vi "2 - Real API list + loop.vi"() -> ()   [LabVIEW 2020]
uses:
  client/client.lvlib
panel:
  out "Array":string[](array[string])
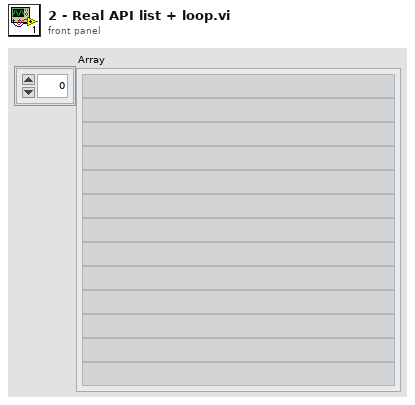
[diagram p1: front panel]
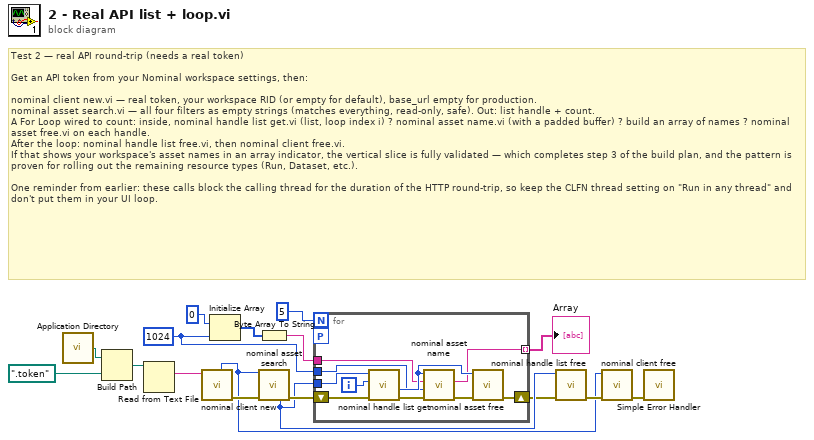
[diagram p0: block diagram]
diagram:
  w7 = 1024
  # "Test 2 — real API round-trip (needs a real token)\n\nGet an API token from your Nominal workspace settings, then:\n\nnominal client new.vi — real token, your workspace RID (or empty for default), base_url empty for production.\nnominal asset search.vi — all four filters as empty strings (matches everything, read-only, safe). Out: list handle + count.\nA For Loop wired to count: inside, nominal handle list get.vi (list, loop index i) ? nominal asset name.vi (with a padded buffer) ? build an array of names ? nominal asset free.vi on each handle.\nAfter the loop: nominal handle list free.vi, then nominal client free.vi.\nIf that shows your workspace's asset names in an array indicator, the vertical slice is fully validated — which completes step 3 of the build plan, and the pattern is proven for rolling out the remaining resource types (Run, Dataset, etc.).\n\nOne reminder from earlier: these calls block the calling thread for the duration of the HTTP round-trip, so keep the CLFN thread setting on \"Run in any thread\" and don't put them in your UI loop."
  n1 = call <vilib>:"Application Directory.vi"() -> ("Application Directory"=w5:path)
  n2 = Build Path(base path=w5, name or relative path=path ".token") -> (appended path=w3:path)
  n3 = Read from Text File(file (use dialog)=w3) -> (text=w2:string)  [unwired: 3 in, 3 out]
  n4 = call "nominal client new.vi"("token"=w2) -> ("error out"=w16:errorcluster, "out_client out"=w12:i32)  [unwired: 8 in, 1 out]
  n5 = Initialize Array(u8 0, w7) -> (w9:u8[])
  n6 = Byte Array To String(unsigned byte array=w9) -> (string=w8:string)
  n7 = call "nominal asset search.vi"("client"=w12, "error in (no error)"=w16) -> ("out_list out"=w15:i32, "error out"=w17:errorcluster)  [unwired: 10 in, 2 out]
  n8 = for {
    N: 5 -> [_]
    tunnel: w15 -> [w27]
    shift-right: [w21] -> w14
    shift-left: w17 -> [w22]
    tunnel: w8 -> [w20]
    tunnel: w7 -> [w19]
    tunnel: [w18] -> w6 mode=indexing
    workers-P: _ -> [_]
    i -> [w25]
    n9 = call "nominal handle list get.vi"("error in (no error)"=w22, "index"=w25, "list"=w27) -> ("error out"=w23:errorcluster, "out_handle out"=w26:i32)  [unwired: 6 in, 1 out]
    n10 = call "nominal asset name.vi"("error in (no error)"=w23, "cap"=w19, "buf"=w20, "asset"=w26) -> ("error out"=w24:errorcluster, "buf out"=w18:string)  [unwired: 4 in, 2 out]
    n11 = call "nominal asset free.vi"("error in (no error)"=w24, "asset"=w26) -> ("error out"=w21:errorcluster)  [unwired: 8 in, 1 out]
  }
  "Array" <- w6
  n12 = call "nominal handle list free.vi"("error in (no error)"=w14, "list"=w15) -> ("error out"=w13:errorcluster)  [unwired: 8 in, 1 out]
  n13 = call "nominal client free.vi"("error in (no error)"=w13, "client"=w12) -> ("error out"=w11:errorcluster)  [unwired: 8 in, 1 out]
  n14 = call <vilib>:"Simple Error Handler.vi"("error in (no error)"=w11) -> ()  [unwired: 4 in, 5 out]
